vi "NiceTimer.vi"(8 "Wait Duration":dbl=2.0 format="%#_13g", 10 "Reset Timer":bool, 11 "Current time":dbl) -> (0 "Single Event True":bool, 3 "Time's up bubby":bool)   [LabVIEW 2013]
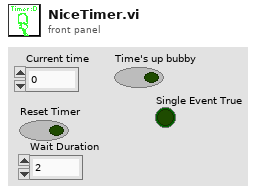
[diagram p1: front panel]
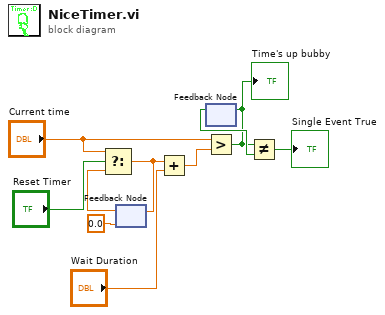
[diagram p0: block diagram]
diagram:
  n1 = feedback #1(0.0 ("FPGA Time")) -> (w5:dbl)
  n2 = Select(t="Current time", s="Reset Timer", f=w5) -> (s? t:f=w6:dbl)
  n3 = feedback-in #1(w6) -> ()
  n4 = Add(x=w6, y="Wait Duration") -> (x+y=w8:dbl)
  n5 = feedback #2() -> (w2:bool)  [unwired: 1 in]
  n6 = Greater?(x="Current time", y=w8) -> (0:w1:bool)
  "Time's up bubby" <- w1
  n7 = feedback-in #2(w1) -> ()
  n8 = Not Equal?(x=w1, y=w2) -> (x != y?=→"Single Event True":bool)
